vi "queues4.vi"() -> ()   [LabVIEW 2018]
doc: "This is the first of two demos using Queues. In this demo, one While loop takes the same role as the first loop in the Notifier example, whilst the second While loop plots data. Here, however, the Wait period in the second (consumer) loop is longer than the producer, and so data builds up over time. Because these are using a Queue, the data is not lost - it merely becomes backlogged."
panel:
  in  "stop 2":bool
  in  "Reset":bool
  out "Count":u32
  in  "Button":bool
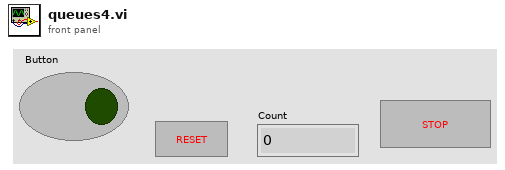
[diagram p1: front panel]
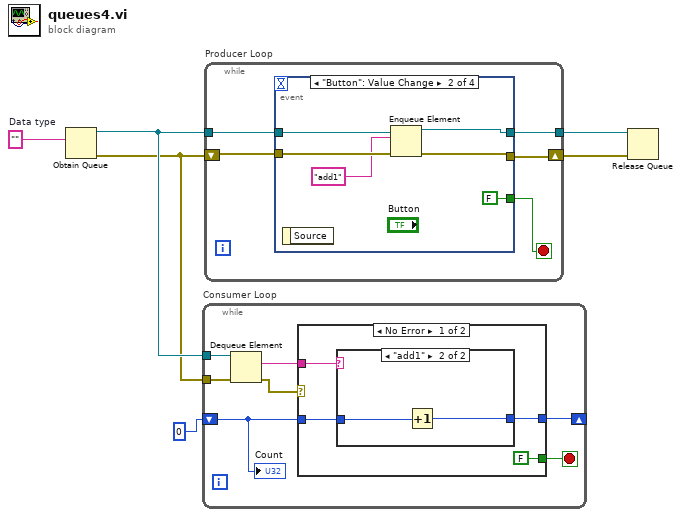
[diagram p0: block diagram]
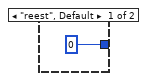
[diagram p2: hidden frame]
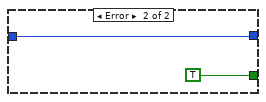
[diagram p3: hidden frame]
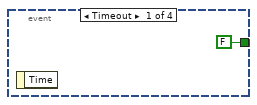
[diagram p4: hidden frame]
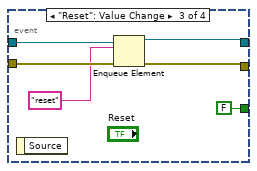
[diagram p5: hidden frame]
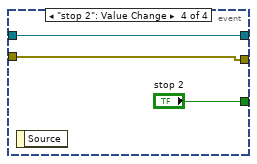
[diagram p6: hidden frame]
diagram:
  w2 = ""  # Data type
  n1 = Obtain Queue(element data type=w2) -> (queue out=w6:refnum<queue>, error out=w3:errorcluster)  [unwired: 4 in, 1 out]
  n2 = while "Consumer Loop" {
    tunnel: w6 -> [w13]
    tunnel: w3 -> [w9]
    shift-right: [w8] -> _
    shift-left: u32 0 -> [w7]
    stop <- w10 stop-if-true
    n3 = Dequeue Element(queue=w13, error in (no error)=w9) -> (element=w11:string, error out=w12:errorcluster)  [unwired: 1 in, 2 out]
    n4 = case shown="No Error" w12 {
      tunnel: w11 -> [w16 _]
      tunnel: [FALSE TRUE] -> w10
      tunnel: w7 -> [w15 w21]
      tunnel: [w14 w21] -> w8
      frame No Error {
        n5 = case shown="\"add1\"" w16 {
          tunnel: w15 -> [_ w20]
          tunnel: [0 w19] -> w14
          frame "reest", Default {
          }
          frame "add1" {
            n6 = Increment(x=w20) -> (x+1=w19:u32)
          }
        }
      }
      frame Error {
      }
    }
    "Count" <- w7
  }
  n7 = while "Producer Loop" {
    tunnel: w6 -> [w27]
    shift-right: [w25] -> w4
    shift-left: w3 -> [w26]
    tunnel: [w24] -> w5
    stop <- w23 stop-if-true
    n8 = event shown="[1] \"Button\": Value Change" {
      selector: _ -> [_ _ _ _]
      dyn-events: _ -> [_ _ _ _]
      timeout: _ -> [_ _ _ _]
      tunnel: w27 -> [_ w32 w38 w43]
      tunnel: w26 -> [_ w34 w40 w42]
      tunnel: [_ w33 w39 w42] -> w25
      tunnel: [_ w31 w37 w43] -> w24
      tunnel: [FALSE ("stop") FALSE ("stop") FALSE ("stop") "stop 2"] -> w23
      event Timeout {
        n9 = event-data() -> ()  [unwired: 1 in, 1 out]
      }
      event "Button": Value Change {
        n10 = event-data() -> ()  [unwired: 1 in, 1 out]
        n11 = Enqueue Element(queue=w32, element="add1", error in (no error)=w34) -> (queue out=w31:refnum<queue>, error out=w33:errorcluster)  [unwired: 1 in, 1 out]
      }
      event "Reset": Value Change {
        n12 = event-data() -> ()  [unwired: 1 in, 1 out]
        n13 = Enqueue Element(queue=w38, element="reset", error in (no error)=w40) -> (queue out=w37:refnum<queue>, error out=w39:errorcluster)  [unwired: 1 in, 1 out]
      }
      event "stop 2": Value Change {
        n14 = event-data() -> ()  [unwired: 1 in, 1 out]
      }
    }
  }
  n15 = Release Queue(queue=w5, error in (no error)=w4) -> ()  [unwired: 1 in, 3 out]
